vi "ExecuteProgram.vi"(8 "error in (no error)":errorcluster, 9 "taskId":i32(ring) items=["TLibrary", "T01", "T02", "T03", "T04", "T05", "T06", "T07", "T08", "T09", "T10", "T11", "T12", "T13", "T14", "T15", "T16", "T17", "T18", "T19", "T20", "T21", "T22", "T23", "T24", "T25", "T26", "T27", "T28", "T29", "T30", "T31"], 10 "program name and path":path, 11 "controller in":refnum<k24>) -> (0 "error out":errorcluster, 2 "success":bool, 3 "controller out":refnum<k24>)   [LabVIEW 2010]
uses:
  c:/aerotech/controller/5.xx.xxx/A3200/pc/labview/2010/bin/Aerotech.A3200.dll
  bin/Aerotech.A3200.dll
  c:/aerotech/controller/5.xx.xxx/A3200/pc/labview/2010/bin/Aerotech.A3200.LabVIEW.dll
  bin/Aerotech.A3200.LabVIEW.dll
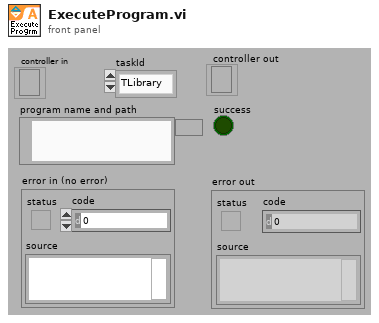
[diagram p1: front panel]
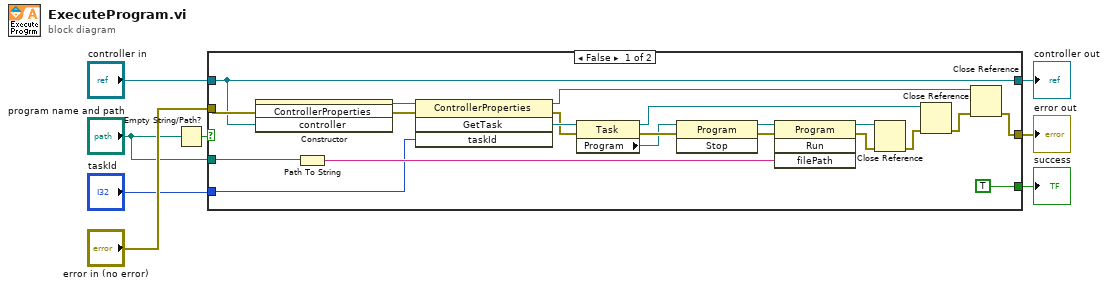
[diagram p0: block diagram]
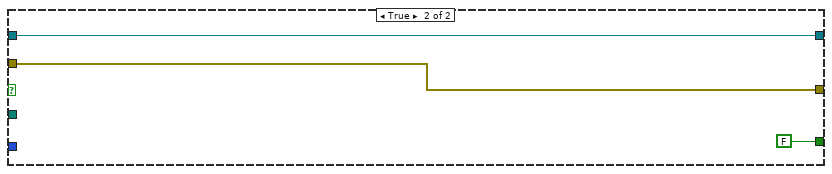
[diagram p2: hidden frame]
diagram:
  n1 = Empty String/Path?(string/path="program name and path") -> (empty?=w5:bool)
  n2 = case shown="False" w5 {
    tunnel: "error in (no error)" -> [w29 w31]
    tunnel: "controller in" -> [w11 w32]
    tunnel: "taskId" -> [w9 _]
    tunnel: [w25 w31] -> w6
    tunnel: "program name and path" -> [w12 _]
    tunnel: [w11 w32] -> w3
    tunnel: [TRUE ("success") FALSE ("success")] -> w2
    frame False {
      n3 = constructor class="ControllerProperties"(error in=w29, "controller"=w11) -> (reference out=w28:refnum<k24>, error out=w27:errorcluster)  [unwired: 2 in, 2 out]
      n4 = Path To String(path=w12) -> (string=w13:string)
      n5 = invoke class="ControllerProperties" method="GetTask"(reference=w28, error in=w27, "taskId"=w9) -> (reference out=w26:refnum<k24>, error out=w20:errorcluster, "GetTask"=w21:refnum<k24>)  [unwired: 1 in, 1 out]
      n6 = property class="Task"(reference=w21, error in=w20) -> (reference out=w14:refnum<k24>, error out=w19:errorcluster, "Program"=w17:refnum<k24>)
      n7 = invoke class="Program" method="Stop"(reference=w17, error in=w19) -> (reference out=w16:refnum<k24>, error out=w18:errorcluster)  [unwired: 1 in, 1 out]
      n8 = invoke class="Program" method="Run"(reference=w16, error in=w18, "filePath"=w13) -> (reference out=w22:refnum<k24>, error out=w24:errorcluster)  [unwired: 1 in, 2 out]
      n9 = Close Reference(reference=w22, error in (no error)=w24) -> (error out=w23:errorcluster)
      n10 = Close Reference(reference=w14, error in (no error)=w23) -> (error out=w15:errorcluster)
      n11 = Close Reference(reference=w26, error in (no error)=w15) -> (error out=w25:errorcluster)
    }
    frame True {
    }
  }
  "error out" <- w6
  "controller out" <- w3
  "success" <- w2
